vi "Create New.vi"(8 "error in (no error)":errorcluster, 10 "Invocation Request ID":u64) -> (0 "error out":errorcluster, 3 "Invocation Request out":refnum<class "Invocation Request ID.lvclass">)   [LabVIEW 2021, in "wamplv.lvlib" / "Invocation Request ID.lvclass"]
uses:
  Invocation Request ID.lvclass
  Invocation Request ID.lvclass/Invocation Request ID.ctl
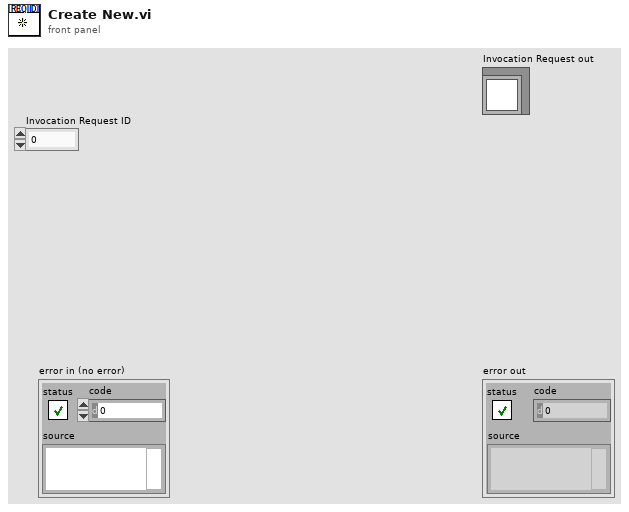
[diagram p1: front panel]
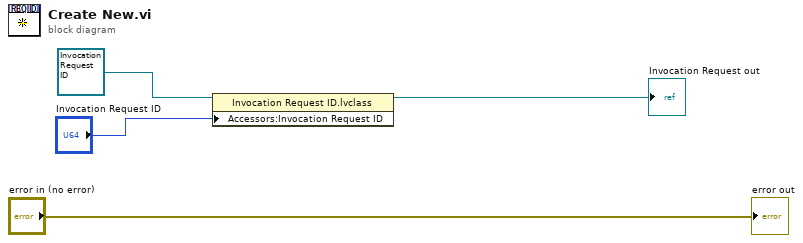
[diagram p0: block diagram]
diagram:
  n1 = property class="Invocation Request ID.lvclass"(reference=refnum<class "Invocation Request ID.lvclass"> refnum, "Accessors:Invocation Request ID"="Invocation Request ID") -> (reference out=→"Invocation Request out":refnum<class "Invocation Request ID.lvclass">)  [unwired: 1 in, 1 out]
  "error out" <- "error in (no error)"
